vi "Read.vi"(8 "error in (no error)":errorcluster, 11 "NI Vision Camera Device in":refnum<class "NI Vision Camera Device.lvclass">) -> (0 "error out":errorcluster, 1 "timed out?":bool=TRUE, 2 "Data":u8[][](array[numeric]), 3 "NI Vision Camera Device out":refnum<class "NI Vision Camera Device.lvclass">)   [LabVIEW 2014, in "NI Vision Camera Device.lvclass"]
uses:
  NI Vision Camera Device.lvclass
  <vilib>/Utility/error.llb/DialogType.ctl
  NI Vision Camera Device.lvclass/NI Vision Camera Device.ctl
  <vilib>/vision/driver/NI_Vision_Acquisition_Software.lvlib
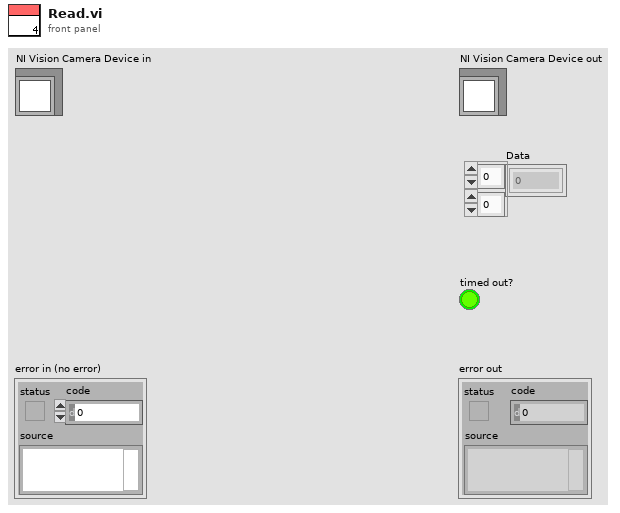
[diagram p1: front panel]
types:
  T1 = typedef "DialogType.ctl" = u16
  T2 = typedef "Image Type" = u32
  T3 = typedef "IMAQdx.ctl" = refnum<k21>
  T4 = typedef "IMAQ Image.ctl" = refnum<image>
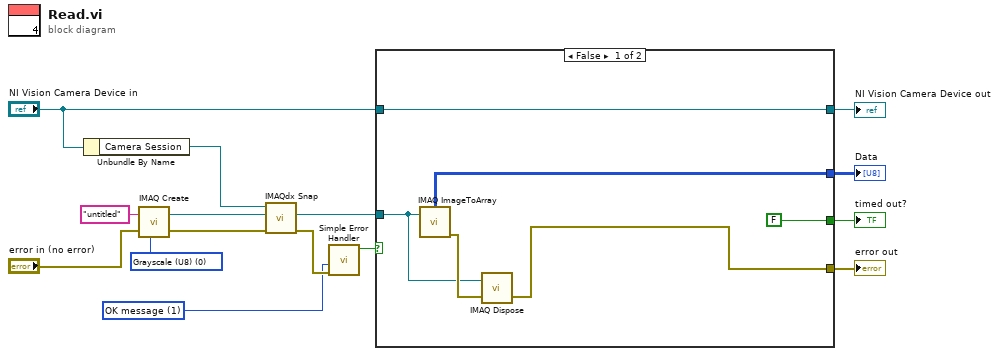
[diagram p0: block diagram]
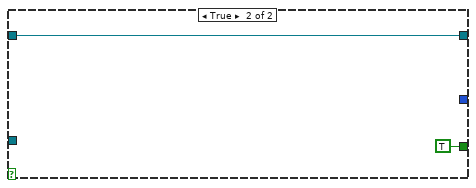
[diagram p2: hidden frame]
diagram:
  w3 = T1 1 items=["no dialog", "OK message", "continue or stop message", "OK message + warnings", "continue/stop + warnings"] ("type of dialog (OK msg:1)")
  w7 = T2 0 items=["Grayscale (U8)", "Grayscale (I16)", "Grayscale (SGL)", "Complex (CSG)", "RGB (U32)", "HSL (U32)", "RGB (U64)", "Grayscale (U16)"] ("Image Type")
  n1 = Unbundle By Name("NI Vision Camera Device in") -> ("Camera Session"=w12:T3)
  n2 = call "IMAQ Create"("Image Name"="untitled", "Image Type"=w7, "error in (no error)"="error in (no error)") -> ("New Image"=w10:T4, "error out"=w8:errorcluster)  [unwired: 2 in]
  n3 = call <vilib>:"IMAQdx Snap.vi"("error in"=w8, "Image In"=w10, "Session In"=w12) -> ("error out"=w4:errorcluster, "Image Out"=w6:T4)  [unwired: 6 in, 1 out]
  n4 = call <vilib>:"Simple Error Handler.vi"("type of dialog (OK msg:1)"=w3, "error in (no error)"=w4) -> ("error?"=w2:bool)  [unwired: 3 in, 4 out]
  n5 = case shown="False" w2 {
    tunnel: "NI Vision Camera Device in" -> [w16 w22]
    tunnel: [w16 w22] -> w14
    tunnel: [w18 _] -> w13
    tunnel: w6 -> [w20 _]
    tunnel: [FALSE ("timed out?") TRUE ("timed out?")] -> w5
    tunnel: [w17 _] -> w1
    frame False {
      n6 = call "IMAQ ImageToArray"("Image"=w20) -> ("error out"=w21:errorcluster, "Image Pixels (U8)"=w17:u8[][])  [unwired: 3 in, 3 out]
      n7 = call "IMAQ Dispose"("Image"=w20, "error in (no error)"=w21) -> ("error out"=w18:errorcluster)  [unwired: 4 in]
    }
    frame True {
    }
  }
  "error out" <- w13
  "NI Vision Camera Device out" <- w14
  "timed out?" <- w5
  "Data" <- w1
